vi "Raster_2d_pass_reference.vi"(2 "Save File path":path, 3 "Save?":bool=TRUE, 5 "task in":refnum<k21>, 6 "error in":errorcluster, 7 "Update Rate (Hz)":dbl=100.0, 8 "Y Parameters":T1={"Number of Y Steps"=200, "Max Y (V)"=2.0, "Min Y (V)"=-2.0}, 9 "X Parameters":T2={"Number of X Steps"=200, "Max X (V)"=2.0, "Min X (V)"=-2.0}) -> (0 "error out":errorcluster, 1 "Intensity Graph":dbl[][](graph), 4 "task out":refnum<k21>)   [LabVIEW 2011]
uses:
  <vilib>/DAQmx/write.llb/DAQmx Write (Analog 2D DBL NChan NSamp).vi
  <vilib>/DAQmx/read.llb/DAQmx Read (Counter 1D U32 1Chan NSamp).vi
  <vilib>/DAQmx/create/channels.llb/DAQmx Create Channel (AO-Voltage-Basic).vi
  <vilib>/DAQmx/configure/timing.llb/DAQmx Timing (Sample Clock).vi
  <vilib>/DAQmx/miscellaneous.llb/DAQmx Fill In Error Info.vi
  Program Files/National Instruments/LabVIEW 2011/resource/objmgr/daqmx.rc
panel:
  out "TotalSampPerChanAcquired":dbl
  out "Output:":dbl[][](graph)
  in  "stop":bool
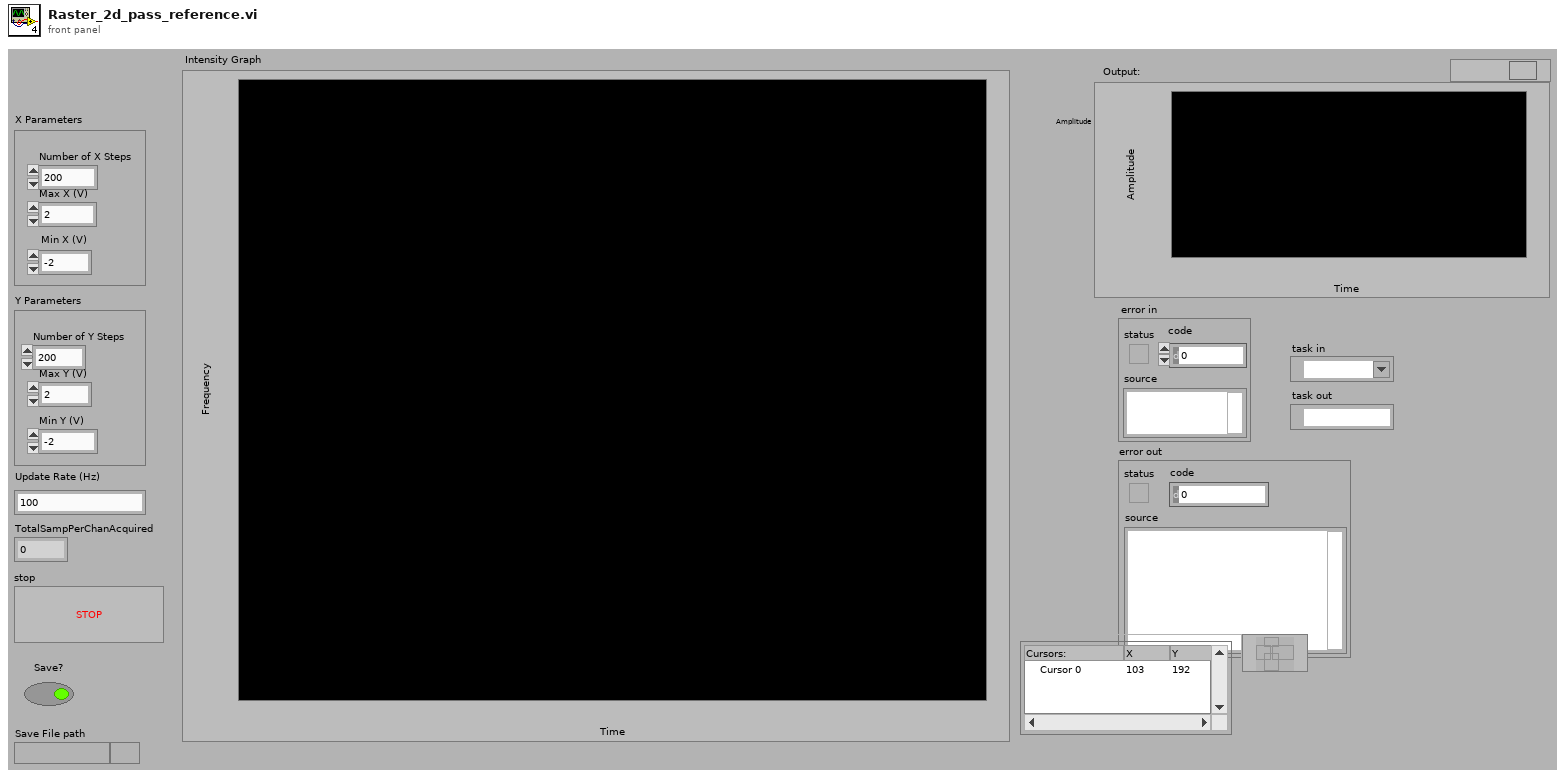
[diagram p1: front panel]
types:
  T1 = cluster{"Number of Y Steps":i32, "Max Y (V)":dbl, "Min Y (V)":dbl}
  T2 = cluster{"Number of X Steps":i32, "Max X (V)":dbl, "Min X (V)":dbl}
  T3 = typedef "imagedata.ctl" = cluster{"image type":i32, "image depth":i32, "image":u8[], "mask":u8[], "colors":u32[], "Rectangle":cluster{"left":i16, "top":i16, "right":i16, "bottom":i16}}
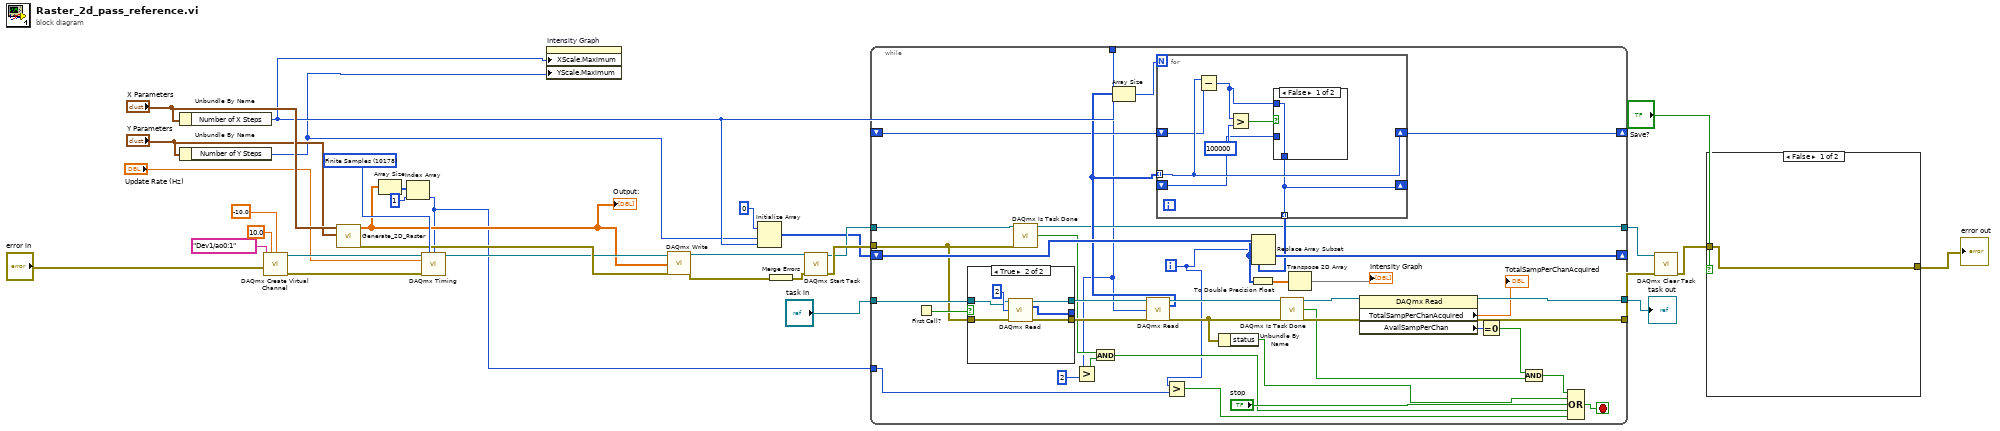
[diagram p0: block diagram]
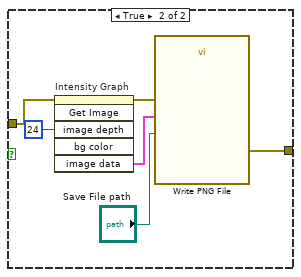
[diagram p2: hidden frame]
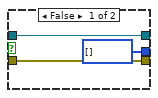
[diagram p4: hidden frame]
diagram:
  w26 = 10178 items=["Finite Samples"=10178, "Continuous Samples"=10123, "Hardware Timed Single Point"=12522] ("sample mode")
  n1 = Unbundle By Name("X Parameters") -> ("Number of X Steps"=w5:i32)
  n2 = Unbundle By Name("Y Parameters") -> ("Number of Y Steps"=w4:i32)
  n3 = call-poly <vilib>:"DAQmx Create Virtual Channel.vi"("maximum value"=10.0, "minimum value"=-10.0, "physical channels"=tag "Dev1/ao0:1", "error in"="error in") -> ("task out"=w32:refnum<k21>, "error out"=w31:errorcluster)  [unwired: 5 in, 5 out]
  n4 = call "Generate_2D_Raster.vi"("Y Parameters"="Y Parameters", "X Parameters"="X Parameters") -> ("error IO"=w20:errorcluster, "Array"=w14:dbl[][])  [unwired: 1 in, 7 out]
  "Output:" <- w14
  n5 = Array Size(array=w14) -> (size(s)=w13:i32[])
  n6 = Index Array(array=w13, index=1) -> (element=w11:i32)
  n7 = call-poly <vilib>:"DAQmx Timing.vi"("task/channels in"=w32, "sample mode"=w26, "samples per channel"=w11, "rate"="Update Rate (Hz)", "error in"=w31) -> ("task out"=w15:refnum<k21>)  [unwired: 2 in, 8 out]
  n8 = property on="Intensity Graph" class="IntGraph (strict)"("XScale.Maximum"=w5, "YScale.Maximum"=w4) -> ()  [unwired: 2 in, 2 out]
  n9 = call-poly <vilib>:"DAQmx Write.vi"("task/channels in"=w15, "data"=w14, "error in"=w20) -> ("task out"=w29:refnum<k21>, "error out"=w21:errorcluster)  [unwired: 1 in, 10 out]
  n10 = Initialize Array(u32 0, w4, w5) -> (w16:u32[][])
  n11 = Merge Errors(w21) -> (w22:errorcluster)
  n12 = call <vilib>:"DAQmx Start Task.vi"("task/channels in"=w29, "error in"=w22) -> ("task out"=w27:refnum<k21>, "error out"=w28:errorcluster)  [unwired: 12 out]
  n13 = while {
    tunnel: w27 -> [w43]
    tunnel: w28 -> [w41]
    tunnel: [w42] -> w25
    tunnel: w5 -> [w37]
    shift-right: [w65] -> _
    shift-left: w16 -> [w66]
    tunnel: w11 -> [w34]
    tunnel: [w61] -> w2
    tunnel: [w62] -> w1
    shift-right: [w47] -> _
    shift-left: _ -> [w46]
    tunnel: "task in" -> [w44]
    i -> [w35]
    stop <- w70 stop-if-true
    n14 = First Call?() -> (First Call?: T/F=w67:bool)
    n15 = case shown="True" w67 {
      tunnel: [w81 w88] -> w69
      tunnel: [w82 w87] -> w68
      tunnel: w41 -> [w82 w86]
      tunnel: w44 -> [w81 w84]
      tunnel: [u32[] [] ("data") w83] -> _
      frame False {
      }
      frame True {
        n16 = call-poly <vilib>:"DAQmx Read.vi"("task/channels in"=w84, "number of samples per channel"=2, "error in"=w86) -> ("task out"=w88:refnum<k21>, "data"=w83:u32[], "error out"=w87:errorcluster)  [unwired: 10 out]
      }
    }
    n17 = call <vilib>:"DAQmx Is Task Done.vi"("task/channels in"=w43, "error in"=w41) -> ("task out"=w42:refnum<k21>, "task done?"=w40:bool)  [unwired: 11 in, 1 out]
    n18 = Greater?(x=w37, y=2) -> (0:w39:bool)
    n19 = And(x=w40, y=w39) -> (x .and. y?=w36:bool)
    n20 = call-poly <vilib>:"DAQmx Read.vi"("task/channels in"=w69, "number of samples per channel"=w37, "error in"=w68) -> ("task out"=w63:refnum<k21>, "data"=w49:u32[], "error out"=w54:errorcluster)  [unwired: 1 in, 9 out]
    n21 = Array Size(array=w49) -> (size(s)=w50:i32)
    n22 = for {
      N: w50 -> [_]
      tunnel: w49 -> [w77] mode=indexing
      shift-right: [w77] -> w47
      shift-left: w46 -> [w76]
      tunnel: [w72] -> w48 mode=indexing
      shift-right: [w72] -> _
      shift-left: _ -> [w71]
      n23 = Subtract(x=w77, y=w76) -> (x-y=w73:u32)
      n24 = Greater?(x=w73, y=u32 100000) -> (0:w74:bool)
      n25 = case shown="False" w74 {
        tunnel: w73 -> [w78 _]
        tunnel: [w78 w79] -> w72
        tunnel: w71 -> [_ w79]
        frame False {
        }
        frame True {
        }
      }
    }
    n26 = Greater?(x=w35, y=w34) -> (0:w33:bool)
    n27 = Unbundle By Name(w54) -> ("status"=w52:bool)
    n28 = Replace Array Subset(array=w66, new element=w48, index (row)=w35) -> (w65:u32[][])  [unwired: 1 in]
    n29 = To Double Precision Float(number=w65) -> (double precision float=w64:dbl[][])
    n30 = call <vilib>:"DAQmx Is Task Done.vi"("task/channels in"=w63, "error in"=w54) -> ("task out"=w60:refnum<k21>, "task done?"=w57:bool, "error out"=w59:errorcluster)  [unwired: 11 out]
    n31 = Transpose 2D Array(2D array=w64) -> (transposed array=→"Intensity Graph":dbl[][])
    n32 = property class="DAQmx Read"(reference=w60, error in=w59) -> (reference out=w62:refnum<k21>, error out=w61:errorcluster, "TotalSampPerChanAcquired"=→"TotalSampPerChanAcquired":dbl, "AvailSampPerChan"=w56:u32)
    n33 = Equal To 0?(x=w56) -> (x = 0?=w55:bool)
    n34 = Compound Arithmetic op=AND(w55, w57) -> (w51:bool)
    n35 = Compound Arithmetic op=OR(w51, w52, "stop", w36, w33) -> (w70:bool)
  }
  "task out" <- w1
  n36 = call <vilib>:"DAQmx Clear Task.vi"("task in"=w25, "error in"=w2) -> ("error out"=w10:errorcluster)  [unwired: 13 out]
  n37 = case shown="False" "Save?" {
    tunnel: w10 -> [w89 w93]
    tunnel: [w89 w95] -> w9
    frame False {
    }
    frame True {
      n38 = invoke on="Intensity Graph" class="IntGraph (strict)" method="Get Image"(error in=w93, "image depth"=24 ("Image Depth")) -> (error out=w92:errorcluster, "image data"=w91:T3)  [unwired: 4 in, 4 out]
      n39 = call <vilib>:"Write PNG File.vi"("error in (no error)"=w92, "image data"=w91, "path to PNG file"="Save File path") -> ("error out"=w95:errorcluster)  [unwired: 7 in, 1 out]
    }
  }
  "error out" <- w9
